vi "Configure Data Logger.vi"(6 "file name":string, 7 "decimal separator":u16(ring) items=["comma", "point"], 8 "error in (no error)":errorcluster, 9 "interval":u16(ring) items=["1 s", "10 s", "30 s", "60 s", "value change >= 1 %", "value change >= 5 %"], 10 "action":u16(ring) items=["stop", "start", "clear"], 11 "VGC in":refnum<class "PL Inficon VGC.lvclass">) -> (0 "error out":errorcluster, 1 "interval":u16(ring) items=["1 s", "10 s", "30 s", "60 s", "value change >= 1 %", "value change >= 5 %"], 2 "action":u16(ring) items=["stop", "start", "clear"], 3 "VGC out":refnum<class "PL Inficon VGC.lvclass">, 4 "file name":string, 5 "decimal separator":u16(ring) items=["comma", "point"])   [LabVIEW 2015, in "PL Inficon VGC.lvclass"]
doc: "Configures data logger."
uses:
  PL Inficon VGC.lvclass
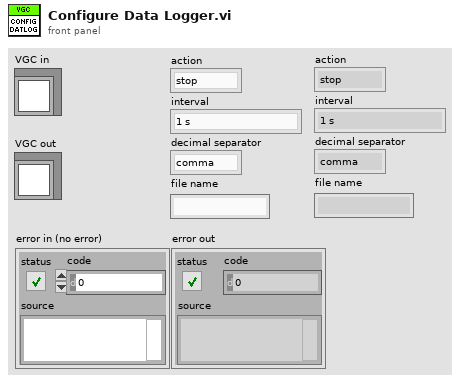
[diagram p1: front panel]
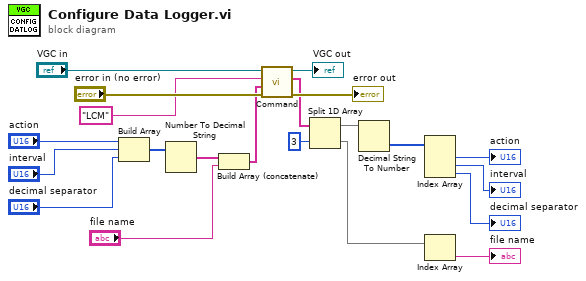
[diagram p0: block diagram]
diagram:
  n1 = Build Array("action", "interval", "decimal separator") -> (w11:u16[])
  n2 = Number To Decimal String(number=w11) -> (decimal integer string=w17:string[])  [unwired: 1 in]
  n3 = Build Array (concatenate)(w17, "file name") -> (w16:string[])
  n4 = call "Command.vi"("error in (no error)"="error in (no error)", "parameters"=w16, "command"="LCM" ("format string"), "VGC in"="VGC in") -> ("error out"=→"error out":errorcluster, "response data"=w9:string[], "VGC out"=→"VGC out":refnum<class "PL Inficon VGC.lvclass">)  [unwired: 5 in]
  n5 = Split 1D Array(array=w9, index=3) -> (first subarray=w7:string[], second subarray=w5:string[])
  n6 = Decimal String To Number(string=w7) -> (number=w6:i32[])  [unwired: 2 in, 1 out]
  n7 = Index Array(array=w6) -> (element #1=→"action":i32, element #2=→"interval":i32, element #3=→"decimal separator":i32)  [unwired: 3 in]
  n8 = Index Array(array=w5) -> (element=→"file name":string)  [unwired: 1 in]
